vi "Set Identifier.vi"(8 "error in (no error)":errorcluster, 10 "Identifier":u32=1, 11 "CAN Frame in":refnum<class "CAN Frame.lvclass">) -> (0 "error out":errorcluster, 3 "CAN Frame out":refnum<class "CAN Frame.lvclass">)   [LabVIEW 2023, in "CAN Frame.lvclass"]
uses:
  CAN Frame.lvclass
  CAN Frame.lvclass/CAN Frame.ctl
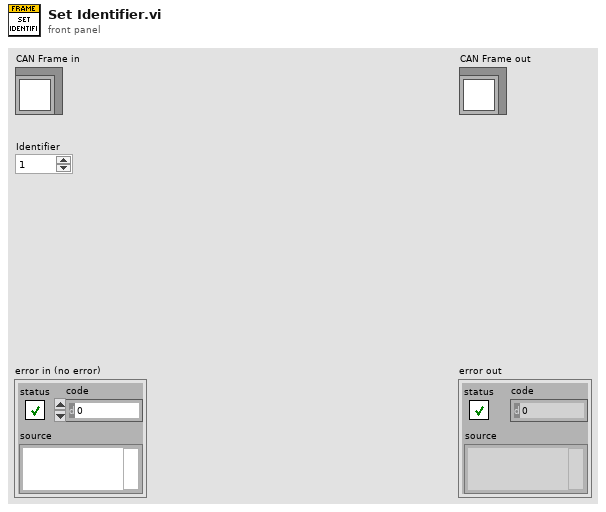
[diagram p1: front panel]
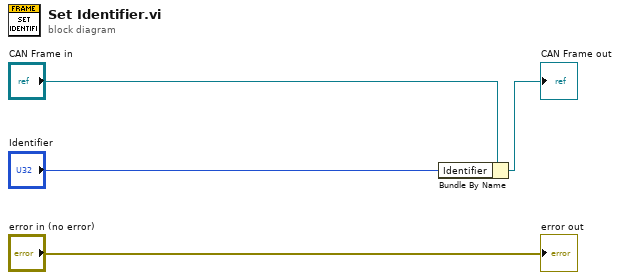
[diagram p0: block diagram]
diagram:
  n1 = Bundle By Name(cluster="CAN Frame in", "Identifier"="Identifier") -> (→"CAN Frame out":refnum<class "CAN Frame.lvclass">)
  "error out" <- "error in (no error)"
